vi "synergia Main.vi"() -> ()   [LabVIEW 2013]
doc: "This template is for the Queued Message Handler design pattern.\n\nThe Event Handling Loop generates messages based on user interface actions.\n\nThe Message Handling Loop processes messages generated by the Event Handling Loop, or by other messages. The messages are string values, so new messages can be added easily to the Message Cases case structure in the Message Handling Loop. Each message cluster can also provide an optional value for Message Data, which is a variant that can be converted to whatever message-specific data is required."
uses:
  Bluetooth/Bluetooth status.ctl
panel:
  out "Bluetooth status":T1
  in  "Right Button":bool
  in  "Left Button":bool
  in  "Backward Button":bool
  in  "Forward Button":bool
  in  "Stop Button":bool
  in  "Stop Bluetooth Button":bool
  in  "Bluetooth Connect Button":bool
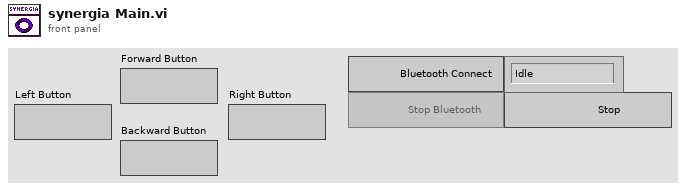
[diagram p1: front panel]
types:
  T1 = typedef "Bluetooth status.ctl" = enum16{"Idle", "Connected"}
  T2 = enum8{"Enabled", "Disabled", "Disabled and Grayed Out"}
  T3 = typedef "eventvkey.ctl" = enum16{"ASCII", "Enter", "Return", "Shift", "Ctrl", "Alt", "Cmd", "Opt", "Caps", "NumLock", "Clear", "Break", "Up", "Down", "Left", "Right", "Insert", "Delete", "Home", "End", "PageUp", "PageDown", "Escape", "Help", "Pause", "ScrollLock", "F1", "F2", "F3", "F4", "F5", "F6", "F7", "F8", "F9", "F10", "F11", "F12", "F13", "F14", "F15", "F16", "F17", "F18", "F19", "F20", "F21", "F22", "F23", "F24", "Play", "VolumeUp", "VolumeDown", "Mute", "Two Byte Char"}
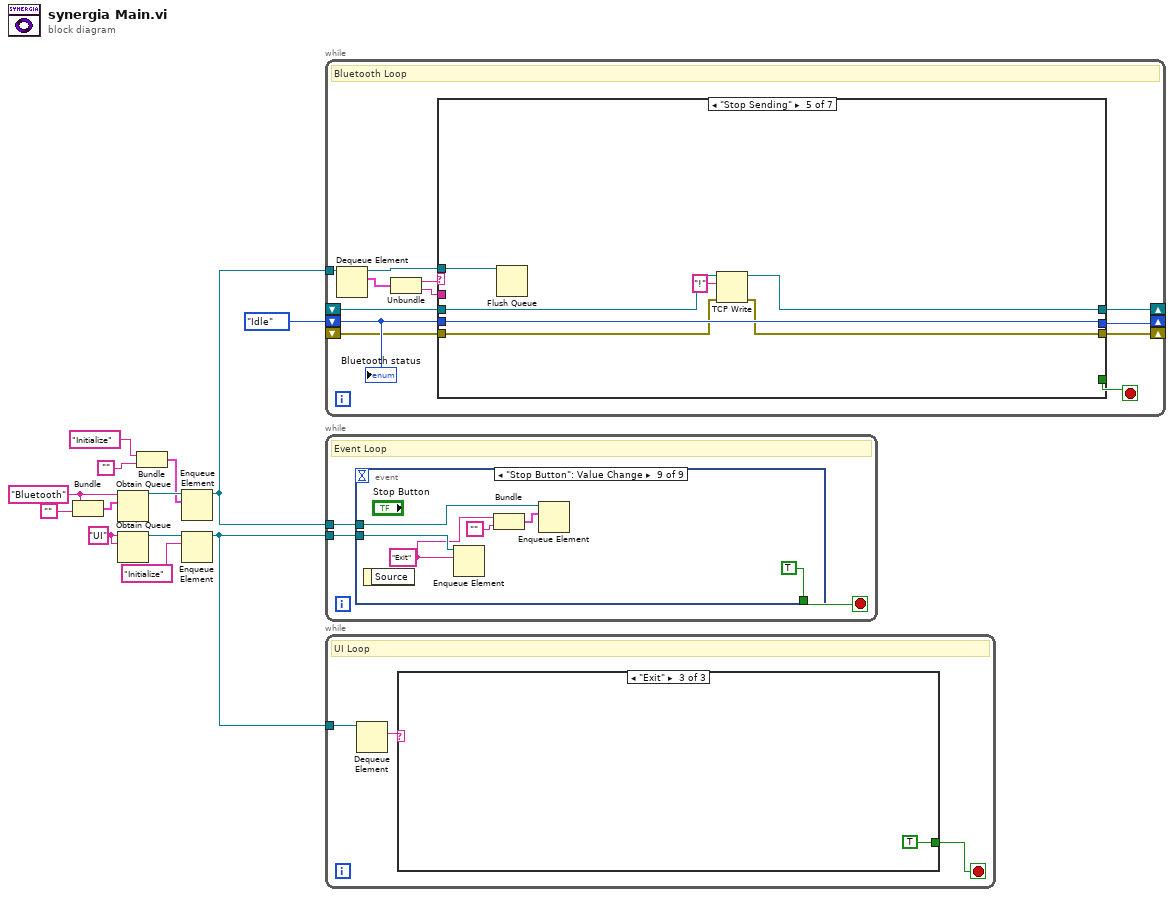
[diagram p0: block diagram]
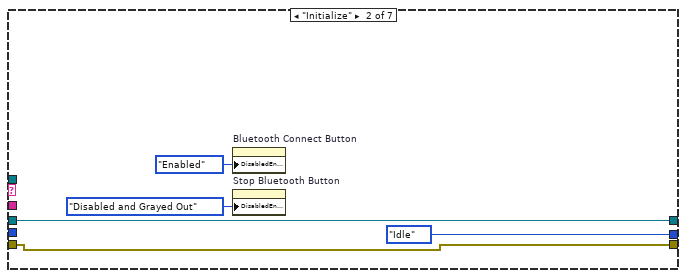
[diagram p3: hidden frame]
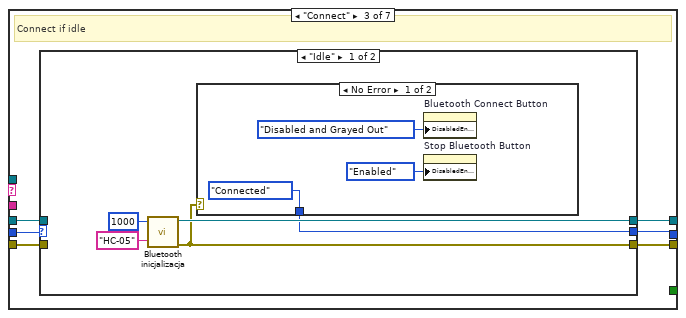
[diagram p4: hidden frame]
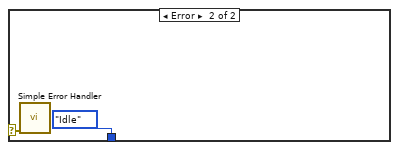
[diagram p5: hidden frame]
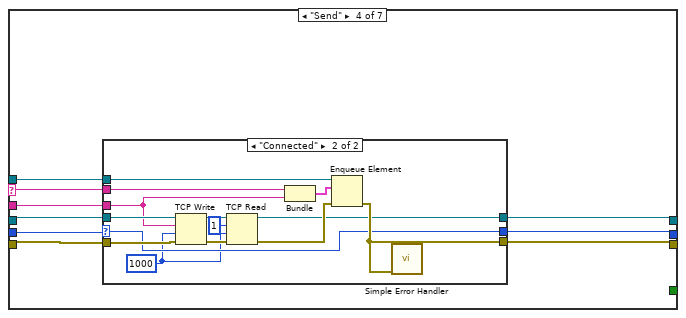
[diagram p7: hidden frame]
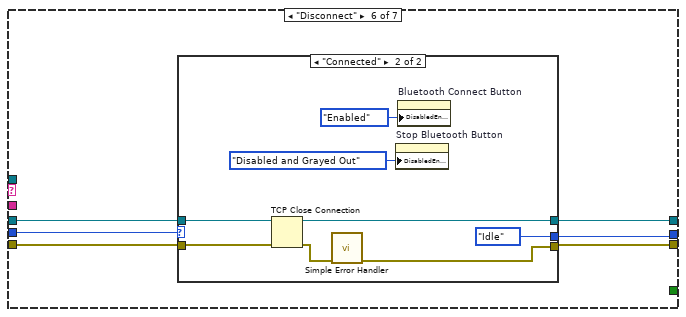
[diagram p9: hidden frame]
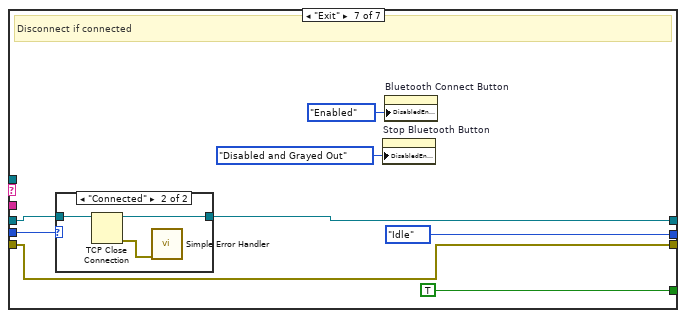
[diagram p11: hidden frame]
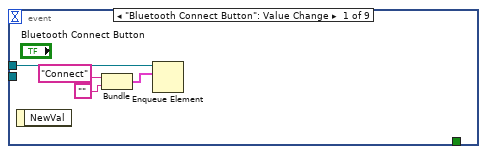
[diagram p15: hidden frame]
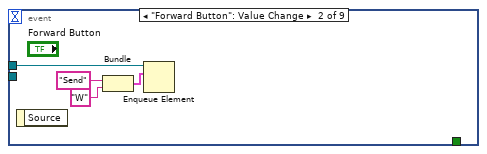
[diagram p16: hidden frame]
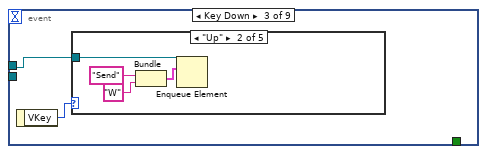
[diagram p17: hidden frame]
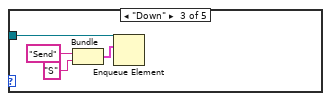
[diagram p19: hidden frame]
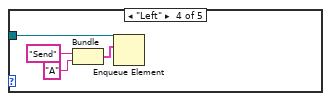
[diagram p20: hidden frame]
diagram:
  w11 = "UI" ("name (unnamed)")
  w3 = "Bluetooth" ("name (unnamed)")
  n1 = Bundle("name (unnamed)"=w3, "") -> (w1:cluster{"name (unnamed)":string, string})  [unwired: 1 in]
  n2 = Obtain Queue(name (unnamed)=w3, element data type=w1) -> (queue out=w13:refnum<queue>)  [unwired: 3 in, 2 out]
  n3 = Obtain Queue(name (unnamed)=w11, element data type=w11) -> (queue out=w10:refnum<queue>)  [unwired: 3 in, 2 out]
  n4 = Bundle("Initialize", "") -> (w4:cluster{string, string})  [unwired: 1 in]
  n5 = Enqueue Element(queue=w13, element=w4) -> (queue out=w8:refnum<queue>)  [unwired: 2 in, 2 out]
  n6 = Enqueue Element(queue=w10, element="Initialize") -> (queue out=w7:refnum<queue>)  [unwired: 2 in, 2 out]
  n7 = while {
    tunnel: w8 -> [w25]
    shift-right: [w23] -> _
    shift-left: Bluetooth_status."Idle" -> [w24]
    shift-right: [w21] -> _
    shift-left: _ -> [w20]
    shift-right: [w19] -> _
    shift-left: _ -> [w18]
    stop <- w22 stop-if-true
    # "Bluetooth Loop"
    n8 = Dequeue Element(queue=w25) -> (queue out=w17:refnum<queue>, element=w16:cluster{"name (unnamed)":string, string})  [unwired: 2 in, 2 out]
    n9 = Unbundle(w16) -> ("name (unnamed)"=w15:string, w14:string)
    n10 = case shown="\"Stop Sending\"" w15 {
      selector: w15 -> [_ _ _ w53 _ _ _]
      tunnel: w24 -> [w28 _ w39 w61 w85 w91 w108]
      tunnel: [w28 Bluetooth_status."Idle" w35 w56 w85 w86 Bluetooth_status."Idle"] -> w23
      tunnel: [_ _ _ _ _ _ TRUE] -> w22
      tunnel: [w27 w32 w38 w57 w82 w87 w106] -> w21
      tunnel: w20 -> [w27 w32 w37 w60 w83 w88 w107]
      tunnel: [w26 w31 w36 w58 w80 w89 w105] -> w19
      tunnel: w18 -> [w26 w31 w34 w59 w81 w90 w105]
      tunnel: w17 -> [_ _ _ w54 w84 _ _]
      tunnel: w14 -> [_ _ _ w55 _ _ _]
      frame Default {
      }
      frame "Initialize" {
        n11 = property on="Bluetooth Connect Button" class="Bool"("DisabledEnum"=T2."Enabled" ("Disabled")) -> ()  [unwired: 2 in, 2 out]
        n12 = property on="Stop Bluetooth Button" class="Bool"("DisabledEnum"=T2."Disabled and Grayed Out" ("Disabled")) -> ()  [unwired: 2 in, 2 out]
      }
      frame "Connect" {
        # "Connect if idle"
        n13 = case shown="\"Idle\"" w39 {
          selector: w39 -> [_ w51]
          tunnel: [w42 w52] -> w38
          tunnel: w37 -> [_ w52]
          tunnel: [w41 w50] -> w36
          tunnel: [w40 w51] -> w35
          tunnel: w34 -> [_ w50]
          frame "Idle" {
            n14 = call "Bluetooth inicjalizacja.vi"("Device Name"="HC-05", "time limit ms (10000)"=1000) -> ("error out"=w41:errorcluster, "Bluetooth Network Connection out"=w42:refnum<k31>)  [unwired: 5 in, 3 out]
            n15 = case shown="No Error" w41 {
              selector: w41 -> [_ w48]
              tunnel: [Bluetooth_status."Connected" Bluetooth_status."Idle"] -> w40
              frame No Error {
                n16 = property on="Bluetooth Connect Button" class="Bool"("DisabledEnum"=T2."Disabled and Grayed Out" ("Disabled")) -> ()  [unwired: 2 in, 2 out]
                n17 = property on="Stop Bluetooth Button" class="Bool"("DisabledEnum"=T2."Enabled" ("Disabled")) -> ()  [unwired: 2 in, 2 out]
              }
              frame Error {
                n18 = call <vilib>:"Simple Error Handler.vi"("error in (no error)"=w48) -> ()  [unwired: 4 in, 5 out]
              }
            }
          }
          frame "Connected", Default {
          }
        }
      }
      frame "Send" {
        n19 = case shown="\"Connected\"" w61 {
          selector: w61 -> [w63 w71]
          tunnel: w60 -> [w64 w78]
          tunnel: w59 -> [w62 w77]
          tunnel: [w62 w75] -> w58
          tunnel: [w64 w65] -> w57
          tunnel: [w63 w71] -> w56
          tunnel: w55 -> [_ w72]
          tunnel: w54 -> [_ w76]
          tunnel: w53 -> [_ w73]
          frame "Idle", Default {
          }
          frame "Connected" {
            w66 = 1000 ("timeout ms (25000)")
            n20 = TCP Write(connection ID=w78, data in=w72, error in (no error)=w77, 9:w66) -> (connection ID out=w70:refnum<k31>, error out=w69:errorcluster)  [unwired: 1 out]
            n21 = TCP Read(connection ID=w70, bytes to read=1, error in (no error)=w69, 9:w66) -> (connection ID out=w65:refnum<k31>, error out=w68:errorcluster)  [unwired: 1 in, 1 out]
            n22 = Bundle(w73, w72) -> (w74:cluster{string, string})  [unwired: 1 in]
            n23 = Enqueue Element(queue=w76, element=w74, error in (no error)=w68) -> (error out=w75:errorcluster)  [unwired: 1 in, 2 out]
            n24 = call <vilib>:"Simple Error Handler.vi"("error in (no error)"=w75) -> ()  [unwired: 4 in, 5 out]
          }
        }
      }
      frame "Stop Sending" {
        n25 = Flush Queue(queue=w84) -> ()  [unwired: 1 in, 3 out]
        n26 = TCP Write(connection ID=w83, data in="!", error in (no error)=w81) -> (connection ID out=w82:refnum<k31>, error out=w80:errorcluster)  [unwired: 1 in, 1 out]
      }
      frame "Disconnect" {
        n27 = case shown="\"Connected\"" w91 {
          selector: w91 -> [w93 _]
          tunnel: w90 -> [w94 w102]
          tunnel: [w94 w97] -> w89
          tunnel: w88 -> [w92 w100]
          tunnel: [w92 w99] -> w87
          tunnel: [w93 Bluetooth_status."Idle"] -> w86
          frame "Idle", Default {
          }
          frame "Connected" {
            n28 = TCP Close Connection(connection ID=w100, error in (no error)=w102) -> (connection ID out=w99:refnum<k31>, error out=w101:errorcluster)  [unwired: 1 in]
            n29 = call <vilib>:"Simple Error Handler.vi"("error in (no error)"=w101) -> ("error out"=w97:errorcluster)  [unwired: 4 in, 4 out]
            n30 = property on="Stop Bluetooth Button" class="Bool"("DisabledEnum"=T2."Disabled and Grayed Out" ("Disabled")) -> ()  [unwired: 2 in, 2 out]
            n31 = property on="Bluetooth Connect Button" class="Bool"("DisabledEnum"=T2."Enabled" ("Disabled")) -> ()  [unwired: 2 in, 2 out]
          }
        }
      }
      frame "Exit" {
        # "Disconnect if connected"
        n32 = case shown="\"Connected\"" w108 {
          tunnel: w107 -> [w111 w113]
          tunnel: [w111 w112] -> w106
          frame "Idle", Default {
          }
          frame "Connected" {
            n33 = TCP Close Connection(connection ID=w113) -> (connection ID out=w112:refnum<k31>, error out=w114:errorcluster)  [unwired: 2 in]
            n34 = call <vilib>:"Simple Error Handler.vi"("error in (no error)"=w114) -> ()  [unwired: 4 in, 5 out]
          }
        }
        n35 = property on="Stop Bluetooth Button" class="Bool"("DisabledEnum"=T2."Disabled and Grayed Out" ("Disabled")) -> ()  [unwired: 2 in, 2 out]
        n36 = property on="Bluetooth Connect Button" class="Bool"("DisabledEnum"=T2."Enabled" ("Disabled")) -> ()  [unwired: 2 in, 2 out]
      }
    }
    "Bluetooth status" <- w24
  }
  n37 = while {
    tunnel: w8 -> [w117]
    tunnel: w7 -> [w116]
    stop <- w115 stop-if-true
    # "Event Loop"
    n38 = event shown="[8] \"Stop Button\": Value Change" {
      selector: _ -> [_ _ _ _ _ _ _ _ _]
      dyn-events: _ -> [_ _ _ _ _ _ _ _ _]
      timeout: _ -> [_ _ _ _ _ _ _ _ _]
      tunnel: w117 -> [w121 w125 w126 w145 w146 w150 w154 w161 w166]
      tunnel: w116 -> [_ _ _ _ _ _ _ _ w165]
      tunnel: [_ _ _ _ _ _ _ _ TRUE] -> w115
      event "Bluetooth Connect Button": Value Change {
        n39 = event-data() -> ()  [unwired: 1 in, 1 out]
        n40 = Bundle("element"="Connect", "") -> (w118:cluster{"element":string, string})  [unwired: 1 in]
        n41 = Enqueue Element(queue=w121, element=w118) -> ()  [unwired: 2 in, 3 out]
      }
      event "Forward Button": Value Change {
        n42 = event-data() -> ()  [unwired: 1 in, 1 out]
        n43 = Bundle("element"="Send", "element"="W") -> (w123:cluster{"element":string, "element":string})  [unwired: 1 in]
        n44 = Enqueue Element(queue=w125, element=w123) -> ()  [unwired: 2 in, 3 out]
      }
      event Key Down {
        n45 = event-data() -> ("VKey"=w127:T3)  [unwired: 1 in]
        n46 = case shown="\"Up\"" w127 {
          tunnel: w126 -> [_ w128 w132 w136 w140]
          frame Default {
          }
          frame "Up" {
            n47 = Bundle("element"="Send", "element"="W") -> (w130:cluster{"element":string, "element":string})  [unwired: 1 in]
            n48 = Enqueue Element(queue=w128, element=w130) -> ()  [unwired: 2 in, 3 out]
          }
          frame "Down" {
            n49 = Bundle("element"="Send", "element"="S") -> (w134:cluster{"element":string, "element":string})  [unwired: 1 in]
            n50 = Enqueue Element(queue=w132, element=w134) -> ()  [unwired: 2 in, 3 out]
          }
          frame "Left" {
            n51 = Bundle("element"="Send", "element"="A") -> (w138:cluster{"element":string, "element":string})  [unwired: 1 in]
            n52 = Enqueue Element(queue=w136, element=w138) -> ()  [unwired: 2 in, 3 out]
          }
          frame "Right" {
            n53 = Bundle("element"="Send", "element"="D") -> (w142:cluster{"element":string, "element":string})  [unwired: 1 in]
            n54 = Enqueue Element(queue=w140, element=w142) -> ()  [unwired: 2 in, 3 out]
          }
        }
      }
      event Key Up {
        n55 = event-data() -> ()  [unwired: 1 in, 1 out]
        n56 = Enqueue Element(queue=w145, element=cluster{"name (unnamed)":string, string} {"name (unnamed)"="Stop Sending", ""}) -> ()  [unwired: 2 in, 3 out]
      }
      event "Backward Button": Value Change {
        n57 = event-data() -> ()  [unwired: 1 in, 1 out]
        n58 = Bundle("element"="Send", "element"="S") -> (w148:cluster{"element":string, "element":string})  [unwired: 1 in]
        n59 = Enqueue Element(queue=w146, element=w148) -> ()  [unwired: 2 in, 3 out]
      }
      event "Left Button": Value Change {
        n60 = event-data() -> ()  [unwired: 1 in, 1 out]
        n61 = Bundle("element"="Send", "element"="A") -> (w152:cluster{"element":string, "element":string})  [unwired: 1 in]
        n62 = Enqueue Element(queue=w150, element=w152) -> ()  [unwired: 2 in, 3 out]
      }
      event "Right Button": Value Change {
        n63 = event-data() -> ()  [unwired: 1 in, 1 out]
        n64 = Bundle("element"="Send", "element"="D") -> (w156:cluster{"element":string, "element":string})  [unwired: 1 in]
        n65 = Enqueue Element(queue=w154, element=w156) -> ()  [unwired: 2 in, 3 out]
      }
      event "Stop Bluetooth Button": Value Change {
        n66 = event-data() -> ()  [unwired: 1 in, 1 out]
        n67 = Bundle("element"="Disconnect", "") -> (w158:cluster{"element":string, string})  [unwired: 1 in]
        n68 = Enqueue Element(queue=w161, element=w158) -> ()  [unwired: 2 in, 3 out]
      }
      event "Stop Button": Value Change {
        w164 = "Exit" ("element")
        n69 = event-data() -> ()  [unwired: 1 in, 1 out]
        n70 = Enqueue Element(queue=w165, element=w164) -> ()  [unwired: 2 in, 3 out]
        n71 = Bundle("element"=w164, "") -> (w162:cluster{"element":string, string})  [unwired: 1 in]
        n72 = Enqueue Element(queue=w166, element=w162) -> ()  [unwired: 2 in, 3 out]
      }
    }
  }
  n73 = while {
    tunnel: w7 -> [w170]
    stop <- w168 stop-if-true
    # "UI Loop"
    n74 = Dequeue Element(queue=w170) -> (element=w169:string)  [unwired: 2 in, 3 out]
    n75 = case shown="\"Exit\"" w169 {
      tunnel: [_ _ TRUE] -> w168
      frame Default {
      }
      frame "Initialize" {
      }
      frame "Exit" {
      }
    }
  }
